vi "Temps and MCs.vi"(8 "error in (no error)":errorcluster, 9 "Motor":i16, 11 "data":waveform(dbl)[](array[waveform])) -> (0 "error out":errorcluster, 1 "Power 1":dbl, 2 "Voltage 1":dbl, 4 "Tank Temp":dbl, 5 "Motor Temp":dbl, 7 "Current 1":dbl)   [LabVIEW 2011]
uses:
  <vilib>/measure/madcrms.llb/Basic Averaged DC-RMS for 1 Chan.vi
  <vilib>/measure/NI_MAPro.lvlib
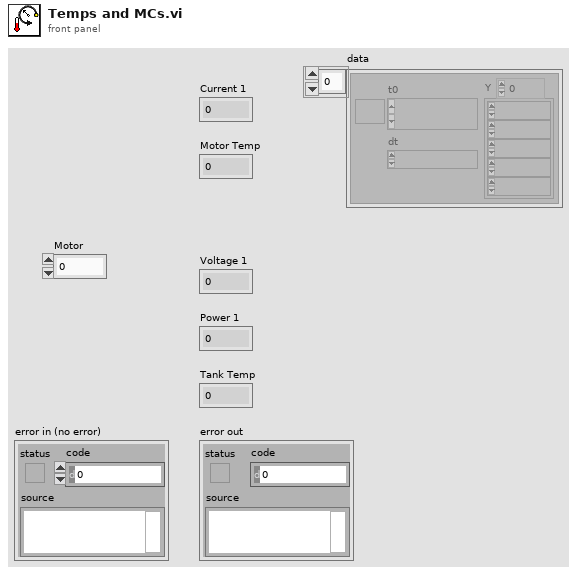
[diagram p1: front panel]
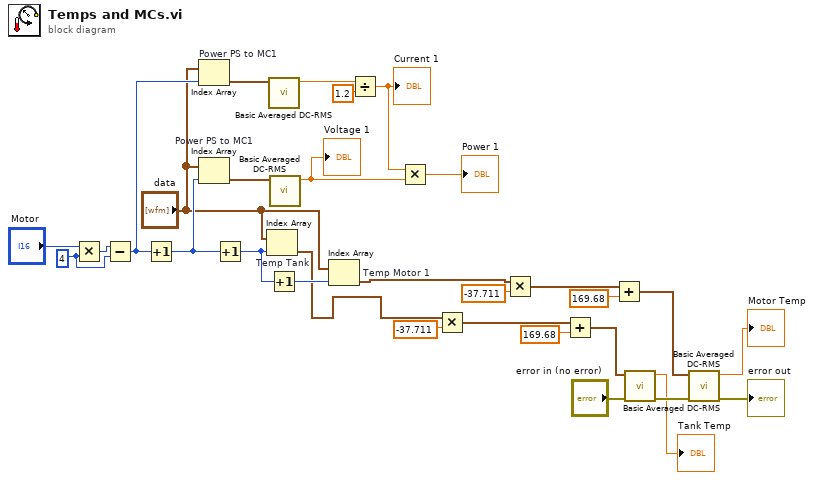
[diagram p0: block diagram]
diagram:
  w3 = i16 4 ("y")
  n1 = Multiply(x="Motor", y=w3) -> (x*y=w4:i16)
  n2 = Subtract(x=w4, y=w3) -> (x-y=w7:i16)
  n3 = Increment(x=w7) -> (x+1=w8:i16)
  n4 = Index Array "Power PS to MC1"(array="data", index=w7) -> (element=w21:waveform(dbl))
  n5 = Index Array "Power PS to MC1"(array="data", index=w8) -> (element=w23:waveform(dbl))
  n6 = Increment(x=w8) -> (x+1=w9:i16)
  n7 = Index Array "Temp Tank"(array="data", index=w9) -> (element=w1:waveform(dbl))
  n8 = call-poly <vilib>:"Basic Averaged DC-RMS.vi"("signal in"=w21) -> ("DC value"=w22:dbl)  [unwired: 7 in, 3 out]
  n9 = Increment(x=w9) -> (x+1=w10:i16)
  n10 = call-poly <vilib>:"Basic Averaged DC-RMS.vi"("signal in"=w23) -> ("DC value"=w24:dbl)  [unwired: 7 in, 3 out]
  "Voltage 1" <- w24
  n11 = Index Array "Temp Motor 1"(array="data", index=w10) -> (element=w2:waveform(dbl))
  n12 = Divide(x=w22, y=1.2) -> (x/y=w19:dbl)
  "Current 1" <- w19
  n13 = Multiply(x=w19, y=w24) -> (x*y=→"Power 1":dbl)
  n14 = Multiply(x=w1, y=-37.711) -> (x*y=w17:waveform(dbl))
  n15 = Multiply(x=w2, y=-37.711) -> (x*y=w14:waveform(dbl))
  n16 = Add(x=w17, y=169.68) -> (x+y=w26:waveform(dbl))
  n17 = Add(x=w14, y=169.68) -> (x+y=w27:waveform(dbl))
  n18 = call-poly <vilib>:"Basic Averaged DC-RMS.vi"("error in (no error)"="error in (no error)", "signal in"=w26) -> ("error out"=w29:errorcluster, "DC value"=→"Tank Temp":dbl)  [unwired: 6 in, 2 out]
  n19 = call-poly <vilib>:"Basic Averaged DC-RMS.vi"("error in (no error)"=w29, "signal in"=w27) -> ("error out"=→"error out":errorcluster, "DC value"=→"Motor Temp":dbl)  [unwired: 6 in, 2 out]
